vi "Previous Scope Selection.vi"(8 "Error In":errorcluster, 10 "Projects":string[](array[string]), 11 "Scope In":refnum<vi>) -> (0 "Error Out":errorcluster, 2 "Previous Selection Index":i32=-1, 3 "Scope Out":refnum<vi>)   [LabVIEW 2017, in "Bookmark Manager.lvlib"]
uses:
  Bookmark Manager.lvlib
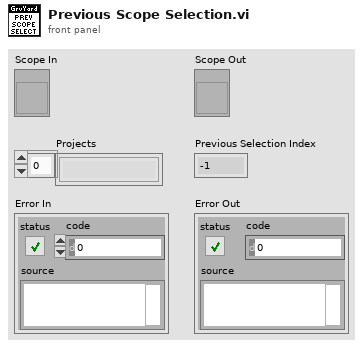
[diagram p1: front panel]
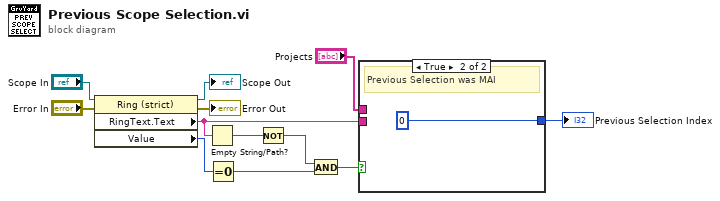
[diagram p0: block diagram]
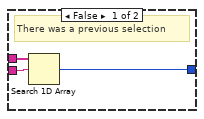
[diagram p2: hidden frame]
diagram:
  n1 = property class="Ring (strict)"(reference="Scope In", error in="Error In") -> (reference out=→"Scope Out":refnum<vi>, error out=→"Error Out":errorcluster, "RingText.Text"=w6:string, "Value"=w9:u16)
  n2 = Empty String/Path?(string/path=w6) -> (empty?=w11:bool)
  n3 = Equal To 0?(x=w9) -> (x = 0?=w8:bool)
  n4 = Not(x=w11) -> (.not. x?=w10:bool)
  n5 = And(x=w10, y=w8) -> (x .and. y?=w7:bool)
  n6 = case shown="True" w7 {
    tunnel: w6 -> [w15 _]
    tunnel: "Projects" -> [w14 _]
    tunnel: [w13 0 ("index of element")] -> w1
    frame False {
      # "There was a previous selection"
      n7 = Search 1D Array(1D array=w14, element=w15) -> (index of element=w13:i32)  [unwired: 1 in]
    }
    frame True {
      # "Previous Selection was MAI"
    }
  }
  "Previous Selection Index" <- w1
